vi "Fetch Measurement (More).vi"(0 "VISA resource name":refnum<visa-resource-name>, 5 "Channel (1: Channel 1)":i32(ring)=1 items=["Channel 1"=1, "Channel 2"=2, "Channel 3"=3, "Channel 4"=4, "Function 1"=5, "Function 2"=6, "Function 3"=7, "Function 4"=8, "Memory 1"=9, "Memory 2"=10, "Memory 3"=11, "Memory 4"=12], 7 "Measurement Function (0: Rise Time)":i32(ring) items=["Rise Time", "Fall Time", "Frequency", "Period", "Voltage RMS(AC)", "Voltage RMS(DC)", "Voltage RMS (AC,cycle)", "Voltage RMS (DC,cycle)", "Voltage Max", "Voltage Min", "Voltage Middle", "Voltage Vpp", "Voltage High", "Voltage Low", "Voltage Average", "Voltage Average (cycle)", "Width Negative", "Width Positive", "Duty Cycle Positive", "Amplitude", "Overshoot", "Preshoot", "Voltage Base", "Voltage Upper", "Time Max", "Time Min", "Color Grade Crossing", "Color Grade Eye Width", "Color Grade Eye Height", "Color Grade Eye Q-Factory", "Color Grade Eye Duty Cycle Distortion(Percent)", "Color Grade Eye Duty Cycle Distortion(Time)", "Color Grade Eye Jitter(PP)", "Color Grade Eye Width(RMS)", "Cycle-cycle Duty Jitter(Rising)", "Cycle-cycle Duty Jitter(Falling)", "Cycle-cycle Jitter(Rising)", "Cycle-cycle Jitter(Falling)", "Cycle-cycle - Width", "Cycle-cycle + Width", "Date Rate", "Unit Interval", "FFT Delta Frequency", "FFT Delta Magnitude", "FFT Frequency", "FFT Magnitude", "Slew Rate", "Area (Entire Display)", "Area(Single Cycle)", "Duty Cycle (Rising)", "Duty Cycle (Falling)"], 11 "error in (no error)":errorcluster) -> (4 "VISA resource name out":refnum<visa-resource-name>, 6 "Measurement":dbl, 15 "error out":errorcluster)   [LabVIEW 2012, in "Agilent 8000 Series.lvlib"]
doc: "Fetches the measurement result for the selected measurement.\n\nNotes:\n\n(1) You must configure the appropriate reference levels before you call this VI to take measurement.\n\n(2) You configure the low, mid, and high references either by calling the Configure Reference Levels.vi.\n\n(3) This VI does not check the instrument status. Typically, you call this VI only in a sequence of calls to other low-level driver VIs. The sequence performs one operation. You use the low-level VIs to optimize one or more aspects of interaction with the instrument. If you want to check the instrument status, call the Error-Query.vi at the conclusion of the sequence.\n\n(4)Duty cycle (rising) and Duty cycle (falling) have been added to the Measurement Function ring control. Data Rate and Unit Interval have their own VI which has added functionality."
uses:
  Agilent 8000 Series.lvlib
panel:
  # "Duty Cycle (rising) and \nDuty cycle falling have\nbeen added."
  # "Data Rate and Unit \ninterval have their own\nVI which has more\nfunctionality."
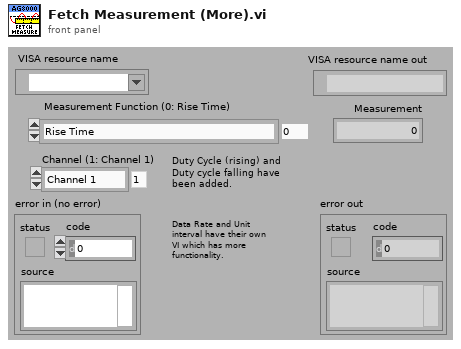
[diagram p1: front panel]
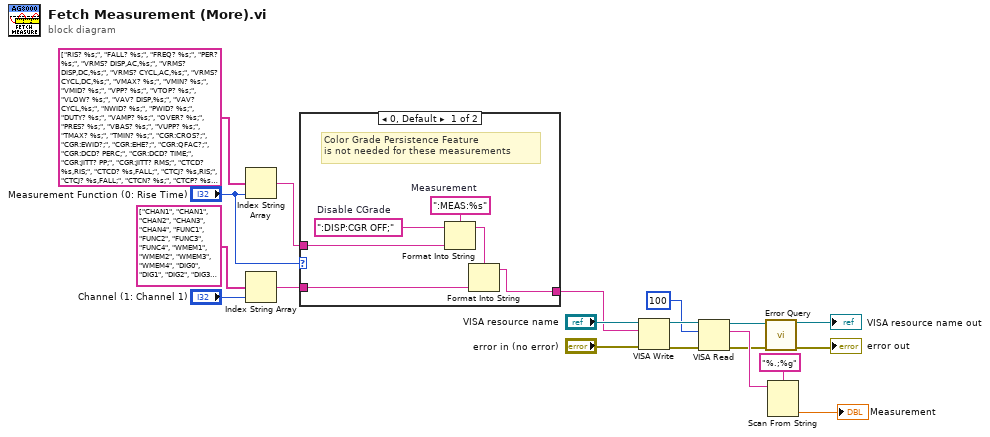
[diagram p0: block diagram]
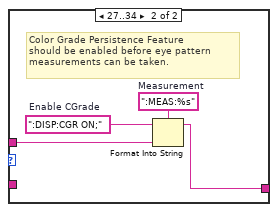
[diagram p2: hidden frame]
diagram:
  n1 = Index String Array(1:"Measurement Function (0: Rise Time)", 2:string[] ["RIS? %s;", "FALL? %s;", "FREQ? %s;", "PER? %s;", "VRMS? DISP,AC,%s;", "VRMS? DISP,DC,%s;", "VRMS? CYCL,AC,%s;", "VRMS? CYCL,DC,%s;", "VMAX? %s;", "VMIN? %s;", "VMID? %s;", "VPP? %s;", "VTOP? %s;", "VLOW? %s;", "VAV? DISP,%s;", "VAV? CYCL,%s;", "NWID? %s;", "PWID? %s;", "DUTY? %s;", "VAMP? %s;", "OVER? %s;", "PRES? %s;", "VBAS? %s;", "VUPP? %s;", "TMAX? %s;", "TMIN? %s;", "CGR:CROS?;", "CGR:EWID?;", "CGR:EHE?;", "CGR:QFAC?;", "CGR:DCD? PERC;", "CGR:DCD? TIME;", "CGR:JITT? PP;", "CGR:JITT? RMS;", "CTCD? %s,RIS;", "CTCD? %s,FALL;", "CTCJ? %s,RIS;", "CTCJ? %s,FALL;", "CTCN? %s;", "CTCP? %s;", "DAT? %s;", "UNIT? %s;", "FFT:DFR? %s;", "FFT:DMAG? %s;", "FFT:FREQ? %s;", "FFT:MAGN? %s;", "SLEW? %s;", "AREA? DISP,%s;", "AREA? CYCL,%s;", "DUTY? %s,RIS;", "DUTY? %s,FALL;"]) -> (0:w15:string)  [unwired: 1 in]
  n2 = Index String Array(1:"Channel (1: Channel 1)", 2:string[] ["CHAN1", "CHAN1", "CHAN2", "CHAN3", "CHAN4", "FUNC1", "FUNC2", "FUNC3", "FUNC4", "WMEM1", "WMEM2", "WMEM3", "WMEM4", "DIG0", "DIG1", "DIG2", "DIG3", "DIG4", "DIG5", "DIG6", "DIG7", "DIG8", "DIG9", "DIG10", "DIG11", "DIG12", "DIG13", "DIG14", "DIG15", "AUX", "LINE"]) -> (0:w5:string)  [unwired: 1 in]
  n3 = case shown="0, Default" "Measurement Function (0: Rise Time)" {
    tunnel: w15 -> [w23 w28]
    tunnel: w5 -> [w21 _]
    tunnel: [w20 w26] -> w4
    frame 0, Default {
      w25 = ":DISP:CGR OFF;"  # Disable CGrade
      w24 = ":MEAS:%s"  # Measurement
      # "Color Grade Persistence Feature\nis not needed for these measurements"
      n4 = Format Into String(format string=w24, initial string=w25, w23) -> (resulting string=w22:string)  [unwired: 1 in, 1 out]
      n5 = Format Into String(format string=w22, w21) -> (resulting string=w20:string)  [unwired: 2 in, 1 out]
    }
    frame 27..34 {
      w27 = ":DISP:CGR ON;"  # Enable CGrade
      w29 = ":MEAS:%s"  # Measurement
      # "Color Grade Persistence Feature\nshould be enabled before eye pattern\nmeasurements can be taken."
      n6 = Format Into String(format string=w29, initial string=w27, w28) -> (resulting string=w26:string)  [unwired: 1 in, 1 out]
    }
  }
  n7 = VISA Write(VISA resource name="VISA resource name", write buffer=w4, error in (no error)="error in (no error)") -> (VISA resource name out=w14:refnum<visa-resource-name>, error out=w13:errorcluster)  [unwired: 1 out]
  n8 = VISA Read(VISA resource name=w14, byte count=u32 100, error in (no error)=w13) -> (VISA resource name out=w12:refnum<visa-resource-name>, read buffer=w10:string, error out=w3:errorcluster)  [unwired: 1 out]
  n9 = call "Error Query.vi"("error in (no error)"=w3, "VISA resource name"=w12) -> ("error out"=→"error out":errorcluster, "VISA resource name out"=→"VISA resource name out":refnum<visa-resource-name>)  [unwired: 6 in, 2 out]
  n10 = Scan From String(format string="%.;%g", input string=w10) -> (output 1=→"Measurement":dbl)  [unwired: 3 in, 3 out]
